vi "clLabview_icon.vi"(11 "vi_lib.lvlib:clLabview.lvclass":refnum<class "clLabview.lvclass">) -> (3 "Icon":picture)   [LabVIEW 2011, in "vi_lib.lvlib" / "clLabview.lvclass"]
uses:
  clLabview.lvclass
  clFileReader/clFileReader.lvclass
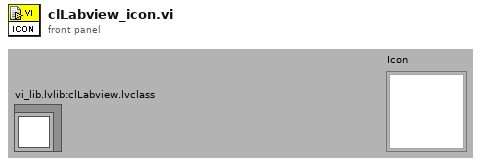
[diagram p1: front panel]
types:
  T1 = typedef "imagedata.ctl" = cluster{"image type":i32, "image depth":i32, "image":u8[], "mask":u8[], "colors":u32[], "Rectangle":cluster{"left":i16, "top":i16, "right":i16, "bottom":i16}}
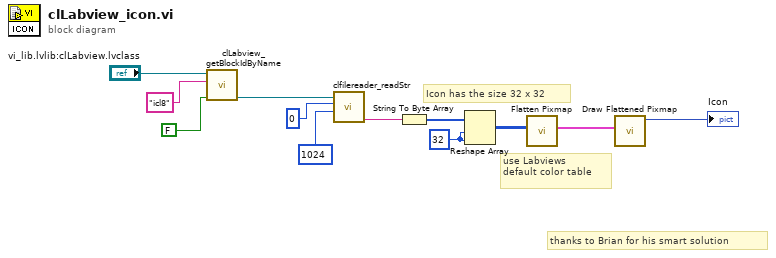
[diagram p0: block diagram]
diagram:
  w1 = 32 ("dimension size")
  # "use Labviews \ndefault color table"
  # "Icon has the size 32 x 32"
  # "thanks to Brian for his smart solution"
  n1 = call "clLabview_getBlockIdByName.vi"("use compression (off)"=FALSE, "Block Name"="icl8", "vi_lib.lvlib:clLabview.lvclass"="vi_lib.lvlib:clLabview.lvclass") -> ("Block Content"=w9:refnum<class "clFileReader.lvclass">)  [unwired: 1 in, 6 out]
  n2 = call "clfilereader_readStr.vi"("size"=u32 1024 ("offset"), "offset"=u32 0 ("size"), "clFileReader.lvclass IN"=w9) -> ("ReadStr - OUT Value"=w4:string)  [unwired: 8 out]
  n3 = String To Byte Array(string=w4) -> (unsigned byte array=w3:u8[])
  n4 = Reshape Array(w3, w1, w1) -> (w2:u8[][])
  n5 = call <vilib>:"Flatten Pixmap.vi"("8-bit pixmap"=w2) -> ("image data"=w5:T1)  [unwired: 5 in, 5 out]
  n6 = call <vilib>:"Draw Flattened Pixmap.vi"("image data"=w5) -> ("new picture"=→"Icon":picture)  [unwired: 1 in, 7 out]
